vi "FTW-Ether-SpawnNewActor-Core.vi"(5 "Configuration":string="{\n  \"Identity\": \"ActorName\",\n  \"DebugEnableInboxLogging\": false,\n  \"DebugEnableJobLogging\": false,\n  \"InboxAddress\": \"inproc://*\",\n  \"DebugShowPanel\": false\n}", 11 "error in":errorcluster, 12 "Register New Addresses":bool=TRUE) -> (4 "FTW Actor Connector":refnum<class "FTW-ActorConnector.lvclass">, 6 "Initialized Response":string, 8 "Instance Inbox Address":string, 15 "error out":errorcluster)   [LabVIEW 2013, in "FTW-Ether.lvclass"]
uses:
  FTW-Ether.lvclass
  Connector/FTW-ActorConnector.lvclass
  JSON/FTW-JSON.lvclass
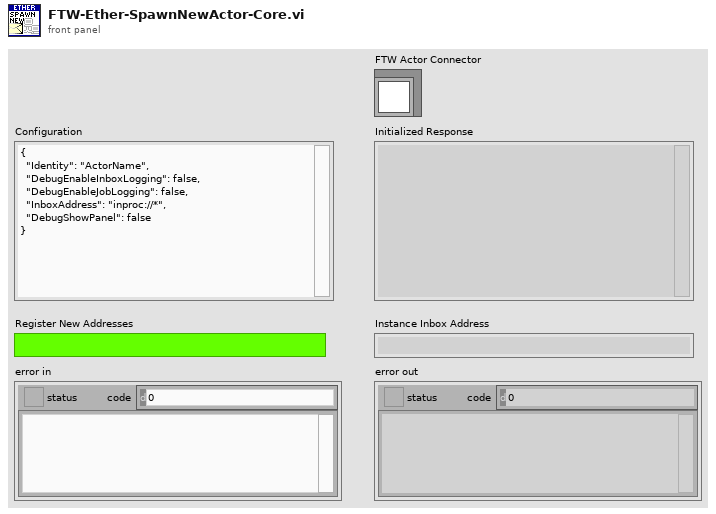
[diagram p1: front panel]
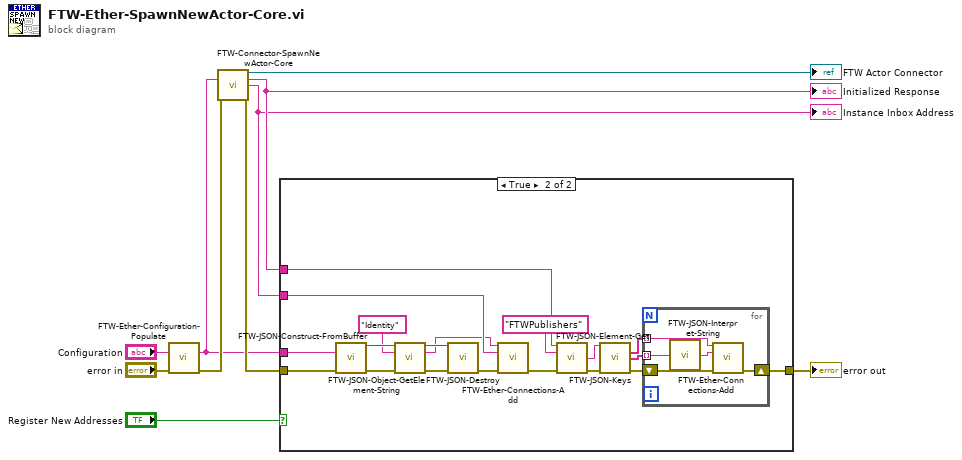
[diagram p0: block diagram]
diagram:
  n1 = call "FTW-Ether-Configuration-Populate.vi"("Configuration String"="Configuration", "error in"="error in") -> ("Filled Configuration String"=w1:string, "error out"=w5:errorcluster)  [unwired: 12 in]
  n2 = call "FTW-Connector-SpawnNewActor-Core.vi"("Configuration"=w1, "error in"=w5) -> ("FTW Actor Connector"=→"FTW Actor Connector":refnum<class "FTW-ActorConnector.lvclass">, "Initialized Response"=w3:string, "Instance Inbox Address"=w2:string, "error out"=w9:errorcluster)  [unwired: 10 in]
  "Initialized Response" <- w3
  "Instance Inbox Address" <- w2
  n3 = case shown="True" "Register New Addresses" {
    tunnel: w9 -> [w11 w30]
    tunnel: [w11 w23] -> w8
    tunnel: w3 -> [_ w20]
    tunnel: w2 -> [_ w19]
    tunnel: w1 -> [_ w18]
    frame False {
    }
    frame True {
      n4 = call "FTW-JSON-Construct-FromBuffer.vi"("JSON String (UTF-8)"=w18, "error in"=w30) -> ("JSON Object"=w17:refnum<class "FTW-JSON.lvclass">, "error out"=w16:errorcluster)  [unwired: 12 in]
      n5 = call "FTW-JSON-Object-GetElement-String.vi"("JSON Object"=w17, "Key"="Identity", "error in"=w16) -> ("JSON Object out"=w13:refnum<class "FTW-JSON.lvclass">, "Value"=w12:string, "error out"=w14:errorcluster)  [unwired: 9 in, 1 out]
      n6 = call "FTW-JSON-Destroy.vi"("JSON Object"=w13, "error in"=w14) -> ("error out"=w29:errorcluster)  [unwired: 13 in]
      n7 = call "FTW-Ether-Connections-Add.vi"("Connection"=w12, "Address"=w19, "error in"=w29) -> ("error out"=w21:errorcluster)  [unwired: 12 in]
      n8 = call "FTW-JSON-Element-Get.vi"("JSON Opject"=w20, "Key"="FTWPublishers", "error in"=w21) -> ("Element"=w27:string, "error out"=w26:errorcluster)  [unwired: 10 in, 1 out]
      n9 = call "FTW-JSON-Keys.vi"("JSON Opject"=w27, "error in"=w26) -> ("Keys"=w25:string[], "Values"=w24:string[], "error out"=w22:errorcluster)  [unwired: 11 in]
      n10 = for {
        tunnel: w25 -> [w32] mode=indexing
        tunnel: w24 -> [w35] mode=indexing
        shift-right: [w33] -> w23
        shift-left: w22 -> [w34]
        n11 = call "FTW-JSON-Interpret-String.vi"("JSON String"=w35) -> ("LabVIEW String"=w31:string)
        n12 = call "FTW-Ether-Connections-Add.vi"("Connection"=w32, "Address"=w31, "error in"=w34) -> ("error out"=w33:errorcluster)  [unwired: 12 in]
      }
    }
  }
  "error out" <- w8
